vi "PantherLAB_CreateControlsIndicators.vi"(9 "Ephemeral Scripting Info":T1, 10 "Event Info":T2 {"timeout (ms)" min=-1 step=1}, 11 "Module Info":T5) -> (0 "error out":errorcluster)   [LabVIEW 2016]
doc: "This is a scripting plugin that uses the same code to create controls and indicators to any node in the block diagram."
uses:
  <vilib>/Delacor/Delacor QMH/Libraries/_Scripting Support/Module Info--cluster.ctl
  <vilib>/Delacor/Delacor QMH/Libraries/_Scripting Support/Module Type--enum.ctl
  <vilib>/Delacor/Delacor QMH/Libraries/_Scripting Support/Event Info (New)--cluster.ctl
  <vilib>/Delacor/Delacor QMH/Libraries/_Scripting Support/Event Type (New)--enum.ctl
  <vilib>/Delacor/Delacor QMH/Libraries/_Scripting Support/Request Scoping--enum.ctl
  <vilib>/Delacor/Delacor QMH/Libraries/_Scripting Support/Ephemeral Scripting Info--cluster.ctl
  <vilib>/Utility/traverseref.llb/TRef TravTarget.ctl
  <resource>/dialog/lvconfig.llb/LV Config Read Boolean.vi
  <resource>/dialog/lvconfig.llb/LV Config Read Numeric (I32).vi
  <vilib>/Delacor/Delacor QMH/Libraries/_Scripting Support/dqmh_lib_DQMH Scripting Support.lvlib
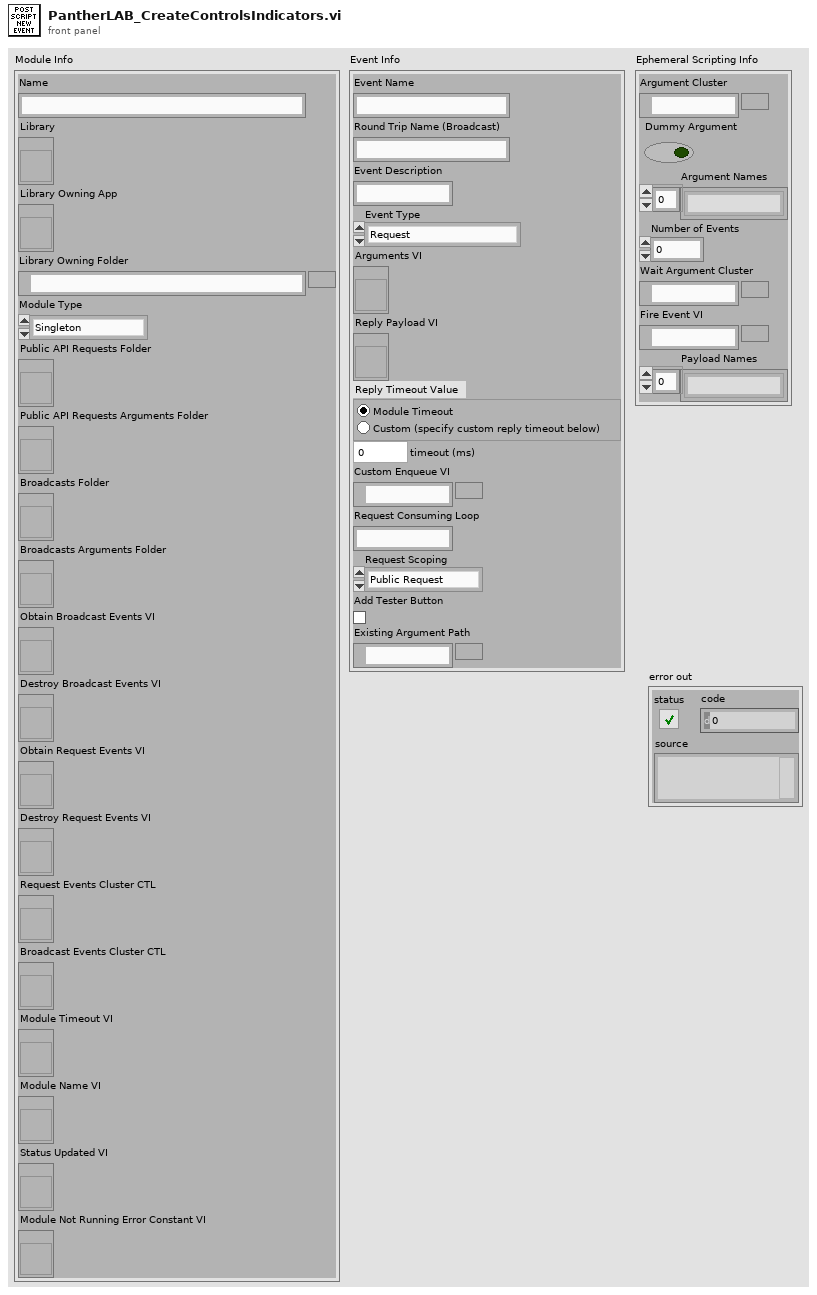
[diagram p1: front panel]
types:
  T1 = typedef "dqmh_lib_DQMH Scripting Support.lvlib/Ephemeral Scripting Info--cluster.ctl" = cluster{"Argument Cluster":path, "Dummy Argument":bool, "Argument Names":string[], "Number of Events":i32, "Wait Argument Cluster":path, "Fire Event VI":path, "Payload Names":string[]}
  T2 = typedef "dqmh_lib_DQMH Scripting Support.lvlib/Event Info (New)--cluster.ctl" = cluster{"Event Name":string, "Round Trip Name (Broadcast)":string, "Event Description":string, "Event Type":T3, "Arguments VI":refnum<vi>, "Reply Payload VI":refnum<vi>, "Reply Timeout Value":enum32{"Module Timeout", "Custom"}, "timeout (ms)":i32, "Custom Enqueue VI":path, "Request Consuming Loop":string, "Request Scoping":T4, "Add Tester Button":bool, "Existing Argument Path":path}
  T3 = typedef "dqmh_lib_DQMH Scripting Support.lvlib/Event Type (New)--enum.ctl" = enum16{"Request", "Broadcast", "Request and Wait for Reply", "Round Trip"}
  T4 = typedef "dqmh_lib_DQMH Scripting Support.lvlib/Request Scoping--enum.ctl" = enum16{"Public Request", "Private Request", "Local Instance"}
  T5 = typedef "dqmh_lib_DQMH Scripting Support.lvlib/Module Info--cluster.ctl" = cluster{"Name":string, "Library":refnum<vi>, "Library Owning App":refnum<vi>, "Library Owning Folder":path, "Module Type":T6, "Public API Requests Folder":refnum<vi>, "Public API Requests Arguments Folder":refnum<vi>, "Broadcasts Folder":refnum<vi>, "Broadcasts Arguments Folder":refnum<vi>, "Obtain Broadcast Events VI":refnum<vi>, "Destroy Broadcast Events VI":refnum<vi>, "Obtain Request Events VI":refnum<vi>, "Destroy Request Events VI":refnum<vi>, "Request Events Cluster CTL":refnum<vi>, "Broadcast Events Cluster CTL":refnum<vi>, "Module Timeout VI":refnum<vi>, "Module Name VI":refnum<vi>, "Status Updated VI":refnum<vi>, "Module Not Running Error Constant VI":refnum<vi>}
  T6 = typedef "dqmh_lib_DQMH Scripting Support.lvlib/Module Type--enum.ctl" = enum16{"Singleton", "Cloneable"}
  T7 = typedef "TRef TravTarget.ctl" = enum16{"FP", "BD", "Other"}
  T8 = enum16{"Controls and Indicators", "Constants and Indicators"}
  T9 = typedef "VariantType.lvlib/Type.ctl" = enum8{"Invalid Type", "Void", "I8", "I16", "I32", "I64", "U8", "U16", "U32", "U64", "Single Float", "Double Float", "Extended Float", "Single Complex", "Double Complex", "Extended Complex", "Enum U8", "Enum U16", "Enum U32", "Enum U64", "Single Float With Unit", "Double Float With Unit", "Extended Float With Unit", "Single Complex with Unit", "Double Complex with Unit", "Extended Complex with Unit", "Boolean", "String", "Path", "Picture", "Tag", "Array", "Cluster", "Variant", "LV Variant", "Waveform", "Timestamp", "Digital Waveform", "Digital Data", "ExpressData", "Refnum", "External Data", "VI", "Poly VI", "LabVIEW Class Instance", "Fixed Point"}
  T10 = typedef "LVRectTypeDef.ctl" = cluster{"Left":i16, "Top":i16, "Right":i16, "Bottom":i16}
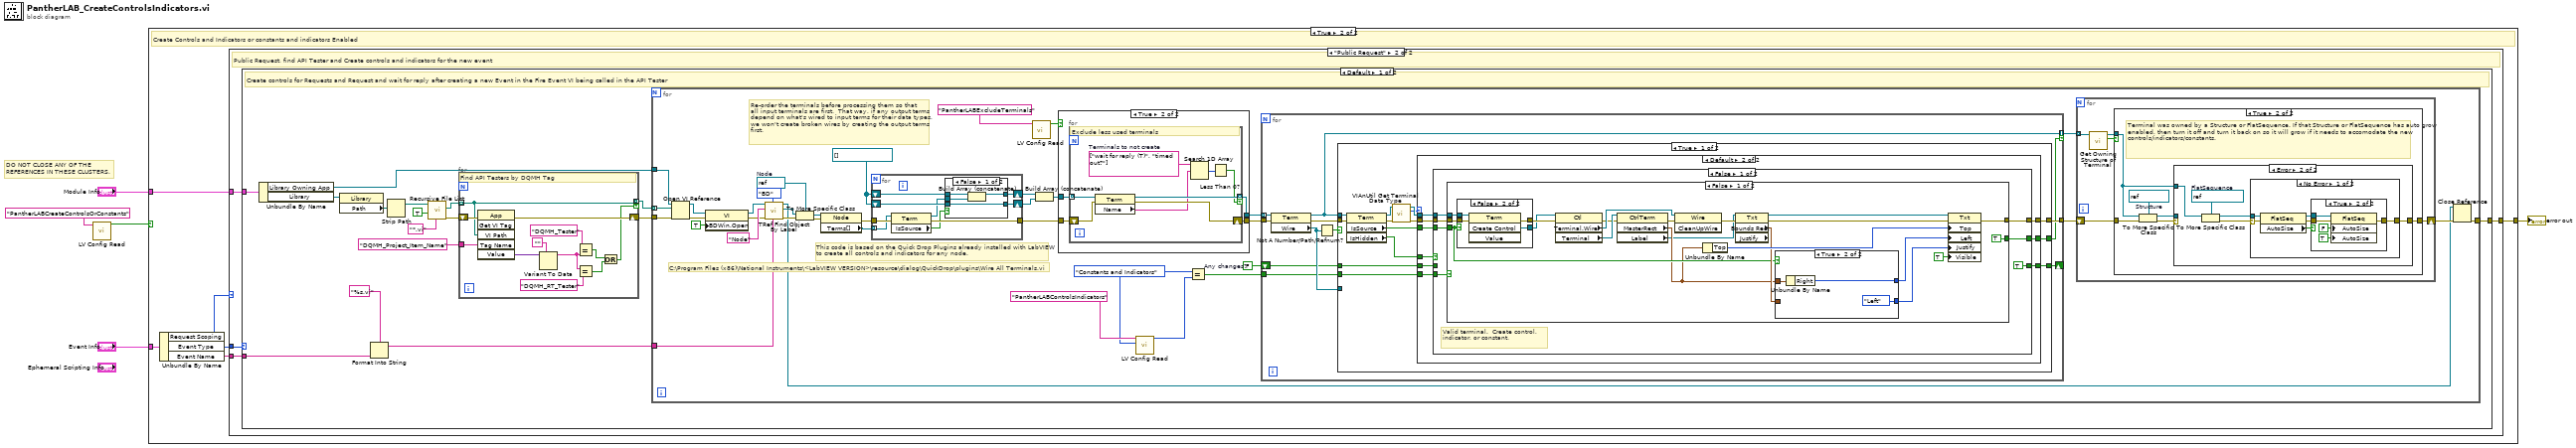
[diagram p0: block diagram]
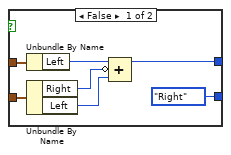
[diagram p6: hidden frame]
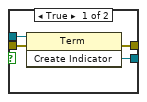
[diagram p7: hidden frame]
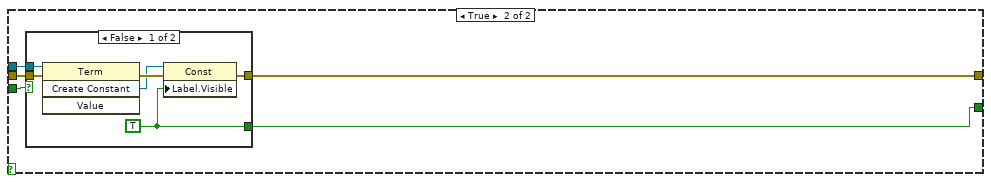
[diagram p8: hidden frame]
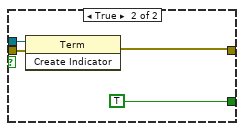
[diagram p9: hidden frame]
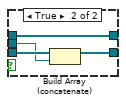
[diagram p12: hidden frame]
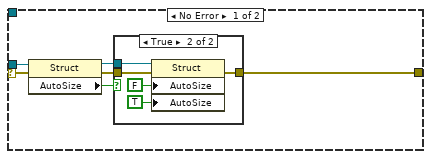
[diagram p14: hidden frame]
diagram:
  # "DO NOT CLOSE ANY OF THE \nREFERENCES IN THESE CLUSTERS."
  n1 = call-poly <resource>:"LV Config Read.vi"("key"="PantherLABCreateControlsOrConstants") -> ("value"=w1:bool)  [unwired: 4 in, 2 out]
  n2 = case shown="True" w1 {
    tunnel: "Module Info" -> [_ w11]
    tunnel: "Event Info" -> [_ w10]
    tunnel: [_ w6] -> w3
    frame False {
      # "Plugin Disabled"
    }
    frame True {
      # "Create Controls and Indicators or constants and indicators Enabled"
      n3 = Unbundle By Name(w10) -> ("Request Scoping"=w7:T4, "Event Type"=w8:T3, "Event Name"=w9:string)
      n4 = case shown="\"Public Request\"" w7 {
        tunnel: w11 -> [_ w15]
        tunnel: w9 -> [_ w14]
        tunnel: w8 -> [_ w13]
        tunnel: [_ w12] -> w6
        frame "Private Request", Default {
          # "This plugin is suited for Public requests"
        }
        frame "Public Request" {
          # "Public Request, find API Tester and Create controls and indicators for the new event"
          n5 = case shown="Default" w13 {
            tunnel: w15 -> [w31 _]
            tunnel: w14 -> [w19 _]
            tunnel: [w16 _] -> w12
            frame Default {
              # "Create controls for Requests and Request and wait for reply after creating a new Event in the Fire Event VI being called in the API Tester"
              n6 = Unbundle By Name(w31) -> ("Library Owning App"=w20:refnum<vi>, "Library"=w30:refnum<vi>)
              n7 = property class="Library"(reference=w30) -> ("Path"=w29:path)  [unwired: 1 in, 2 out]
              n8 = Format Into String(format string="%s.vi", w19) -> (resulting string=w17:string)  [unwired: 2 in, 1 out]
              n9 = Strip Path(path=w29) -> (stripped path=w28:path)  [unwired: 1 out]
              n10 = call <vilib>:"Recursive File List.vi"("pattern"="*.vi", "Continue Recursing on Error? (F)"=TRUE, "Folder Path"=w28) -> ("error out"=w24:errorcluster, "All Files in Dir"=w25:path[])  [unwired: 4 in, 3 out]
              n11 = for {
                tunnel: w25 -> [w33] mode=indexing
                shift-right: [w39] -> w22
                shift-left: w24 -> [w43]
                tunnel: "DQMH_Project_Item_Name" -> [w42]
                tunnel: [w33] -> w21 mode=indexing if=w32
                # "Find API Testers by DQMH Tag"
                n12 = invoke class="App" method="Get VI Tag"(error in=w43, "VI Path"=w33, "Tag Name"=w42) -> (error out=w39:errorcluster, "Value"=w41:variant)  [unwired: 3 in, 4 out]
                n13 = Variant To Data(type="", Variant=w41) -> (data=w36:string)  [unwired: 1 in, 1 out]
                n14 = Equal?(x="DQMH_Tester", y=w36) -> (x = y?=w35:bool)
                n15 = Equal?(x=w36, y="DQMH_RT_Tester" ("x")) -> (x = y?=w34:bool)
                n16 = Or(x=w35, y=w34) -> (x .or. y?=w32:bool)
              }
              n17 = for {
                tunnel: w22 -> [w80]
                tunnel: w21 -> [w79] mode=indexing
                tunnel: w20 -> [w78]
                tunnel: w17 -> [w71]
                tunnel: [w62] -> w16
                w46 = T8."Constants and Indicators" ("x")
                w58 = FALSE  # Any changes?
                w68 = refnum<vi>[] [] ("Terms[]")
                w72 = refnum<vi> refnum  # Node
                # "C:\\Program Files (x86)\\National Instruments\\<LabVIEW VERSION>\\resource\\dialog\\QuickDrop\\plugins\\Wire All Terminals.vi"
                # "This code is based on the Quick Drop Plugins already installed with LabVIEW\nto create all controls and indicators for any node."
                # "Re-order the terminals before processing them so that\nall input terminals are first.  That way, if any output terms\ndepend on what's wired to input terms for their data types,\nwe won't create broken wires by creating the output terms\nfirst."
                n18 = Open VI Reference(application reference (local)=w78, vi path=w79, error in (no error)=w80) -> (vi reference=w52:refnum<vi>, error out=w77:errorcluster)  [unwired: 3 in]
                n19 = property class="VI"(reference=w52, error in=w77, "BDWin.Open"=TRUE ("Block Diagram Window:Open")) -> (reference out=w51:refnum<vi>, error out=w53:errorcluster)
                n20 = call <vilib>:"TRef Find Object By Label.vi"("Label"=w71, "Traverse Target"=TRef_TravTarget."BD", "error in (no error)"=w53, "Class Name"="Node", "VI Ref"=w51) -> ("error out"=w74:errorcluster, "Found Obj Ref"=w73:refnum<vi>, "dup VI Ref"=w61:refnum<vi>)  [unwired: 3 in, 1 out]
                n21 = To More Specific Class(target class=w72, reference=w73, error in=w74) -> (specific class reference=w70:refnum<vi>, error out=w69:errorcluster)
                n22 = property class="Node"(reference=w70, error in=w69) -> (error out=w64:errorcluster, "Terms[]"=w65:refnum<vi>[])  [unwired: 1 out]
                n23 = for {
                  tunnel: w65 -> [w203] mode=indexing
                  shift-right: [w199] -> w67
                  shift-left: w68 -> [w201]
                  shift-right: [w198] -> w66
                  shift-left: w68 -> [w200]
                  tunnel: w64 -> [w204]
                  tunnel: [w202] -> w59
                  n24 = property class="Term"(reference=w203, error in=w204) -> (reference out=w197:refnum<vi>, error out=w202:errorcluster, "IsSource"=w196:bool)
                  n25 = case shown="False" w196 {
                    tunnel: w201 -> [w208 w212]
                    tunnel: w200 -> [w206 w211]
                    tunnel: [w207 w212] -> w199
                    tunnel: [w206 w210] -> w198
                    tunnel: w197 -> [w205 w209]
                    frame False {
                      n26 = Build Array (concatenate)(w208, w205) -> (w207:refnum<vi>[])
                    }
                    frame True {
                      n27 = Build Array (concatenate)(w211, w209) -> (w210:refnum<vi>[])
                    }
                  }
                }
                n28 = call-poly <resource>:"LV Config Read.vi"("key"="PantherLABExcludeTerminals") -> ("value"=w44:bool)  [unwired: 4 in, 2 out]
                n29 = Build Array (concatenate)(w67, w66) -> (w60:refnum<vi>[])
                n30 = case shown="True" w44 {
                  tunnel: w60 -> [w82 w86]
                  tunnel: w59 -> [w81 w85]
                  tunnel: [w81 w84] -> w57
                  tunnel: [w82 w83] -> w56
                  frame False {
                  }
                  frame True {
                    n31 = for {
                      tunnel: w86 -> [w94] mode=indexing
                      tunnel: [w93] -> w83 mode=indexing if=w87
                      shift-right: [w91] -> w84
                      shift-left: w85 -> [w92]
                      w90 = string[] ["wait for reply (T)", "timed out?"]  # Terminals to not create
                      # "Exclude less used terminals"
                      n32 = property class="Term"(reference=w94, error in=w92) -> (reference out=w93:refnum<vi>, error out=w91:errorcluster, "Name"=w89:string)
                      n33 = Search 1D Array(1D array=w90, element=w89) -> (index of element=w88:i32)  [unwired: 1 in]
                      n34 = Less Than 0?(x=w88) -> (x < 0?=w87:bool)
                    }
                  }
                }
                n35 = call-poly <resource>:"LV Config Read.vi"("default value"=w46, "key"="PantherLABControlsIndicators") -> ("value"=w47:i32)  [unwired: 3 in, 2 out]
                n36 = Equal?(x=w46, y=w47) -> (x = y?=w49:bool)
                n37 = for {
                  tunnel: w56 -> [w104] mode=indexing
                  shift-right: [w99] -> _
                  shift-left: w58 -> [w100]
                  tunnel: w49 -> [w97]
                  tunnel: w57 -> [w105]
                  tunnel: [w98] -> w54
                  tunnel: [w96] -> w55 mode=indexing if=w95
                  n38 = property class="Term"(reference=w104, error in=w105) -> (reference out=w96:refnum<vi>, error out=w103:errorcluster, "Wire"=w101:refnum<vi>)
                  n39 = Not A Number/Path/Refnum?(number/path/refnum=w101) -> (NaN/Path/Refnum?=w102:bool)
                  n40 = case shown="True" w102 {
                    tunnel: w103 -> [w119 w194]
                    tunnel: w96 -> [w118 _]
                    tunnel: w101 -> [_ _]
                    tunnel: w100 -> [w115 w195]
                    tunnel: [w117 w195] -> w99
                    tunnel: [w107 w194] -> w98
                    tunnel: w97 -> [w114 _]
                    tunnel: [w106 _] -> w95
                    frame True {
                      n41 = property class="Term"(reference=w118, error in=w119) -> (reference out=w110:refnum<vi>, error out=w112:errorcluster, "IsSource"=w116:bool, "IsHidden"=w113:bool)
                      n42 = call <vilib>:"VIAnUtil Get Terminal Data Type.vi"("error in (no error)"=w112, "Terminal"=w110) -> ("error out"=w111:errorcluster, "Data Type"=w108:T9, "dup  Terminal"=w109:refnum<vi>)  [unwired: 6 in, 1 out]
                      n43 = case shown="Default" w108 {
                        tunnel: [w121 w130] -> w117
                        tunnel: w116 -> [_ w129]
                        tunnel: w109 -> [_ w128]
                        tunnel: [w120 w127] -> w107
                        tunnel: w111 -> [w120 w126]
                        tunnel: w115 -> [w121 w123]
                        tunnel: w114 -> [_ w125]
                        tunnel: w113 -> [_ w124]
                        tunnel: [_ w122] -> w106
                        frame "Invalid Type", "Void" {
                          # "Current terminal is void (like an empty terminal on a subVI).  Do nothing."
                        }
                        frame Default {
                          n44 = case shown="False" w124 {
                            tunnel: [TRUE w192] -> w130
                            tunnel: w129 -> [w136 _]
                            tunnel: w128 -> [w135 _]
                            tunnel: [w134 w193] -> w127
                            tunnel: w126 -> [w133 w193]
                            tunnel: w125 -> [w132 _]
                            tunnel: w123 -> [_ w192]
                            tunnel: [w131 _] -> w122
                            frame False {
                              # "Valid terminal.  Create control, indicator, or constant."
                              n45 = case shown="False" w132 {
                                tunnel: w136 -> [w144 w181]
                                tunnel: w135 -> [w158 w180]
                                tunnel: [w151 w179] -> w134
                                tunnel: w133 -> [w157 w178]
                                tunnel: [TRUE w177] -> w131
                                frame False {
                                n46 = case shown="False" w144 {
                                tunnel: w157 -> [w172 w176]
                                tunnel: w158 -> [w170 w174]
                                tunnel: [w171 w175] -> w155
                                tunnel: [w169 w173] -> w154
                                frame True {
                                n47 = invoke class="Term" method="Create Indicator"(reference=w170, error in=w172) -> (error out=w171:errorcluster, "Create Indicator"=w169:refnum<vi>)  [unwired: 1 in, 1 out]
                                }
                                frame False {
                                n48 = invoke class="Term" method="Create Control"(reference=w174, error in=w176) -> (error out=w175:errorcluster, "Create Control"=w173:refnum<vi>)  [unwired: 2 in, 2 out]
                                }
                                }
                                n49 = property class="Ctl"(reference=w154, error in=w155) -> (error out=w140:errorcluster, "Terminal.Wire"=w153:refnum<vi>, "Terminal"=w142:refnum<vi>)  [unwired: 1 out]
                                n50 = property class="CtrlTerm"(reference=w142, error in=w140) -> (error out=w139:errorcluster, "MasterRect"=w141:T10, "Label"=w138:refnum<vi>)  [unwired: 1 out]
                                n51 = invoke class="Wire" method="CleanUpWire"(reference=w153, error in=w139) -> (error out=w152:errorcluster)  [unwired: 1 in, 2 out]
                                n52 = Unbundle By Name(w141) -> ("Top"=w149:i16)
                                n53 = property class="Txt" props=["Bounds Rect", "Justify"](reference=w138, error in=w152) -> (reference out=w143:refnum<vi>, error out=w148:errorcluster, "Bounds Rect"=w147:T10)  [unwired: 1 out]
                                n54 = case shown="True" w144 {
                                tunnel: w141 -> [w165 w168]
                                tunnel: w147 -> [w163 _]
                                tunnel: [w160 w167] -> w150
                                tunnel: [enum16{"Left", "Center", "Right"}."Right" ("Justification") enum16{"Left", "Center", "Right"}."Left" ("Justification")] -> w146
                                frame False {
                                n55 = Unbundle By Name(w165) -> ("Left"=w164:i16)
                                n56 = Unbundle By Name(w163) -> ("Right"=w162:i16, "Left"=w161:i16)
                                n57 = Compound Arithmetic op=ADD(w164, invert w162, w161) -> (w160:i16)
                                }
                                frame True {
                                n58 = Unbundle By Name(w168) -> ("Right"=w167:i16)
                                }
                                }
                                n59 = property class="Txt"(reference=w143, error in=w148, "Top"=w149, "Left"=w150, "Justify"=w146, "Visible"=TRUE) -> (error out=w151:errorcluster)  [unwired: 1 out]
                                }
                                frame True {
                                n60 = case shown="False" w181 {
                                tunnel: w178 -> [w187 w191]
                                tunnel: w180 -> [w185 w190]
                                tunnel: [w184 w189] -> w179
                                tunnel: [w182 TRUE] -> w177
                                frame False {
                                w182 = TRUE
                                n61 = invoke class="Term" method="Create Constant"(reference=w185, error in=w187) -> (error out=w186:errorcluster, "Create Constant"=w183:refnum<vi>)  [unwired: 2 in, 2 out]
                                n62 = property class="Const"(reference=w183, error in=w186, "Label.Visible"=w182) -> (error out=w184:errorcluster)  [unwired: 1 out]
                                }
                                frame True {
                                n63 = invoke class="Term" method="Create Indicator"(reference=w190, error in=w191) -> (error out=w189:errorcluster)  [unwired: 1 in, 2 out]
                                }
                                }
                                }
                              }
                            }
                            frame True {
                              # "Do not attempt to create inputs/outputs on hidden terminals (like Dynamic Event terms on an Event Structure that aren't showing)"
                            }
                          }
                        }
                      }
                    }
                    frame False {
                      # "Current terminal is wired.  Do nothing."
                    }
                  }
                }
                n64 = for {
                  shift-right: [w213] -> w63
                  shift-left: w54 -> [w214]
                  tunnel: w55 -> [w217] mode=indexing
                  n65 = call <vilib>:"Get Owning Structure of Terminal.vi"("Terminal"=w217) -> ("Terminal Owned by Structure?"=w216:bool, "Owning Structure"=w215:refnum<vi>)  [unwired: 9 in]
                  n66 = case shown="True" w216 {
                    tunnel: w215 -> [_ w219]
                    tunnel: w214 -> [w218 w224]
                    tunnel: [w218 w220] -> w213
                    frame False {
                      # "Terminal was not owned at any point in its hierarchy by a Structure or FlatSequence. This terminal must be on the top-level diagram (or its owning Node is on the top-level diagram)."
                    }
                    frame True {
                      w221 = refnum<vi> refnum  # Structure
                      # "Terminal was owned by a Structure or FlatSequence. If that Structure or FlatSequence has auto grow enabled, then turn it off and turn it back on so it will grow if it needs to accomodate the new controls/indicators/constants."
                      n67 = To More Specific Class(target class=w221, reference=w219, error in=w224) -> (specific class reference=w222:refnum<vi>, error out=w223:errorcluster)
                      n68 = case shown="Error" w223 {
                        selector: w223 -> [w230 _]
                        tunnel: w222 -> [w229 _]
                        tunnel: [w226 w237] -> w220
                        tunnel: w219 -> [_ w240]
                        frame No Error {
                          n69 = property class="Struct"(reference=w229, error in=w230) -> (reference out=w225:refnum<vi>, error out=w227:errorcluster, "AutoSize"=w228:bool)
                          n70 = case shown="True" w228 {
                            tunnel: w227 -> [w231 w235]
                            tunnel: [w231 w234] -> w226
                            tunnel: w225 -> [_ w236]
                            frame False {
                            }
                            frame True {
                              n71 = property class="Struct"(reference=w236, error in=w235, "AutoSize"=FALSE ("AutoSize To Fit Contents?"), "AutoSize"=TRUE ("AutoSize To Fit Contents?")) -> (error out=w234:errorcluster)  [unwired: 1 out]
                            }
                          }
                        }
                        frame Error {
                          w241 = refnum<vi> refnum  # FlatSequence
                          n72 = To More Specific Class(target class=w241, reference=w240) -> (specific class reference=w238:refnum<vi>, error out=w239:errorcluster)  [unwired: 1 in]
                          n73 = case shown="No Error" w239 {
                            selector: w239 -> [w244 _]
                            tunnel: w238 -> [w243 _]
                            tunnel: [w242 _] -> w237
                            frame No Error {
                              n74 = property class="FlatSeq"(reference=w243, error in=w244) -> (reference out=w245:refnum<vi>, error out=w246:errorcluster, "AutoSize"=w247:bool)
                              n75 = case shown="True" w247 {
                                tunnel: w246 -> [w248 w252]
                                tunnel: [w248 w251] -> w242
                                tunnel: w245 -> [_ w253]
                                frame False {
                                }
                                frame True {
                                n76 = property class="FlatSeq"(reference=w253, error in=w252, "AutoSize"=FALSE ("AutoSize To Fit Contents?"), "AutoSize"=TRUE ("AutoSize To Fit Contents?")) -> (error out=w251:errorcluster)  [unwired: 1 out]
                                }
                              }
                            }
                            frame Error {
                            }
                          }
                        }
                      }
                    }
                  }
                }
                n77 = Close Reference(reference=w61, error in (no error)=w63) -> (error out=w62:errorcluster)
              }
            }
            frame "Broadcast" {
              # "If the event is a Broadcast there is no Fire Event VI, do nothing"
            }
          }
        }
      }
    }
  }
  "error out" <- w3
